vi "Edit Lock In (SubVI).vi"(8 "error in (no error)":errorcluster, 11 "Instrument parameters in":T1) -> (0 "error out":errorcluster, 3 "Instrument parameters out":T1)   [LabVIEW 2025, in "MyLockIn.lvlib"]
uses:
  MyLockIn.lvlib
panel:
  in  "Boolean":bool
  in  "Monitor sensitivity":bool
  in  "RESET?":bool
  in  "Auto Reserve":bool
  in  "Auto Phase":bool
  in  "Auto gain":bool
  out "Present value":string
  in  "Set new":bool
  in  "Read":bool
  in  "Select parameter":string(combo)="SENS"
  # "SETTINGS FOR LOCK-IN"
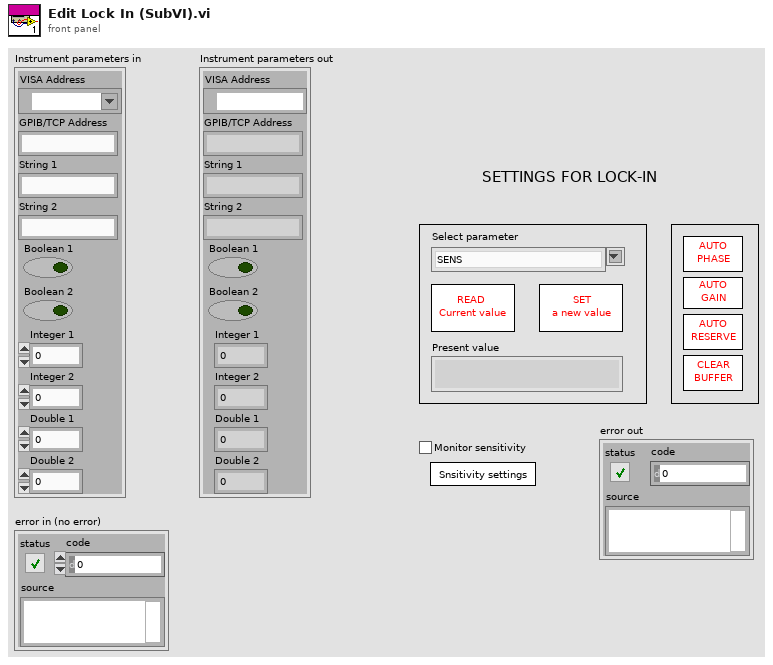
[diagram p1: front panel]
types:
  T1 = cluster{"VISA Address":refnum<visa-resource-name>, "GPIB/TCP Address":string, "String 1":string, "String 2":string, "Boolean 1":bool, "Boolean 2":bool, "Integer 1":i32, "Integer 2":i32, "Double 1":dbl, "Double 2":dbl}
  T2 = typedef "S2DS_Instrument parameters.ctl" = cluster{"VISA Address":refnum<visa-resource-name>, "GPIB/TCP Address":string, "String 1":string, "String 2":string, "Boolean 1":bool, "Boolean 2":bool, "Int 1":i32, "Int 2":i32, "Double 1":dbl, "Double 2":dbl}
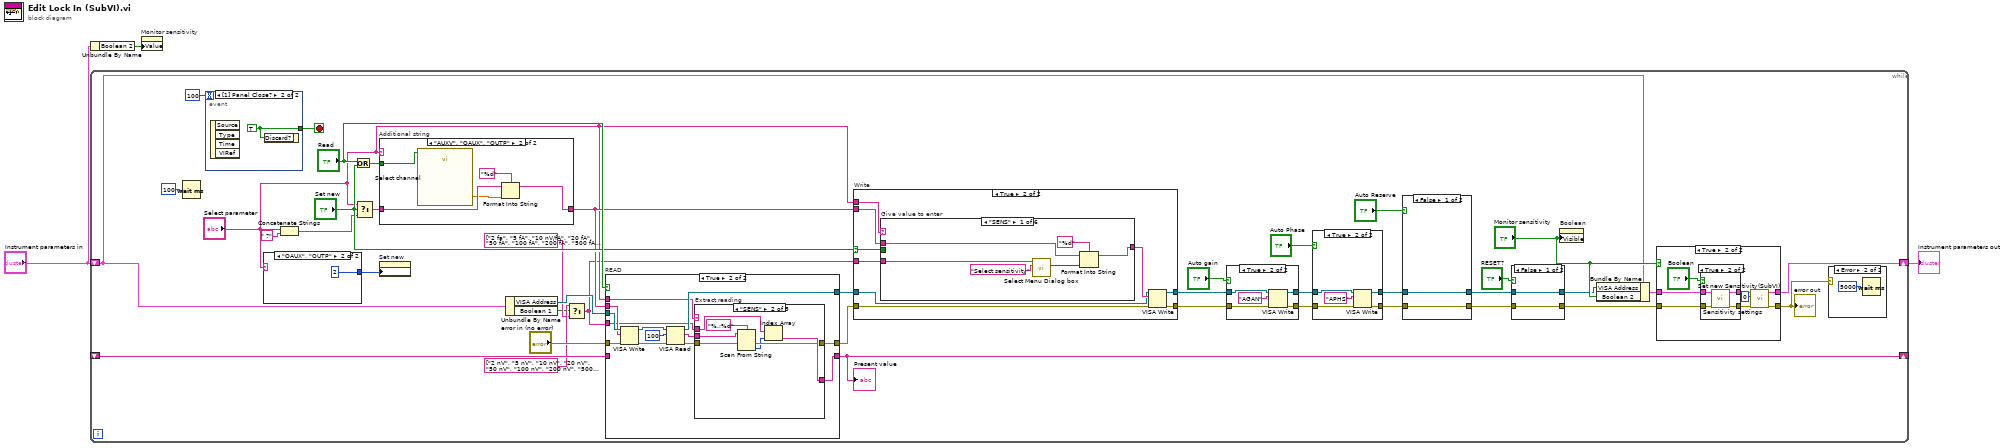
[diagram p0: block diagram]
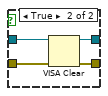
[diagram p4: hidden frame]
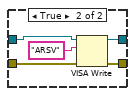
[diagram p5: hidden frame]
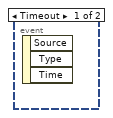
[diagram p9: hidden frame]
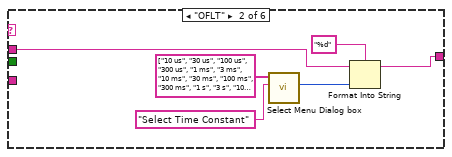
[diagram p11: hidden frame]
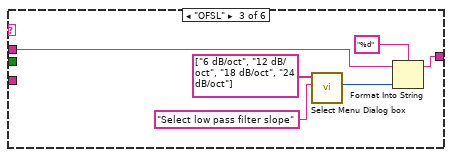
[diagram p12: hidden frame]
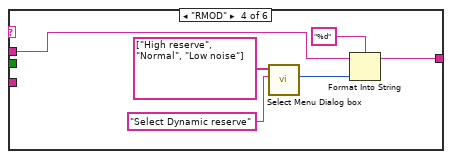
[diagram p13: hidden frame]
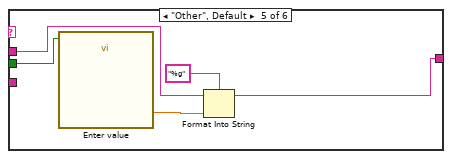
[diagram p14: hidden frame]
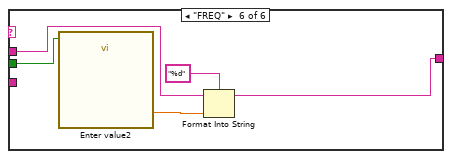
[diagram p15: hidden frame]
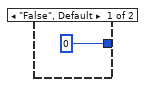
[diagram p16: hidden frame]
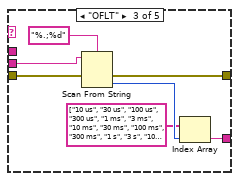
[diagram p19: hidden frame]
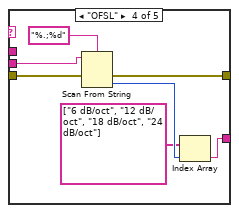
[diagram p20: hidden frame]
diagram:
  n1 = Unbundle By Name("Instrument parameters in") -> ("Boolean 2"=w1:bool)
  n2 = while {
    shift-right: [w37] -> _
    shift-left: _ -> [w36]
    shift-right: [w4] -> w3
    shift-left: "Instrument parameters in" -> [w6]
    stop <- w27 stop-if-true
    n3 = Wait (ms)(milliseconds to wait=u32 100) -> ()  [unwired: 1 out]
    n4 = event shown="[1] Panel Close?" {
      selector: _ -> [_ _]
      dyn-events: _ -> [_ _]
      timeout: 100 -> [_ _]
      tunnel: [_ w89] -> w27
      event Timeout {
        n5 = event-data() -> ()  [unwired: 1 in, 3 out]
      }
      event Panel Close? {
        w89 = TRUE ("Discard?")
        n6 = event-data() -> ()  [unwired: 1 in, 4 out]
        n7 = event-data("Discard?"=w89) -> ()  [unwired: 1 in, 1 out]
      }
    }
    n8 = case shown="\"OAUX\", \"OUTP\"" "Select parameter" {
      tunnel: [0 2] -> w38
      frame "False", Default {
      }
      frame "OAUX", "OUTP" {
      }
    }
    n9 = Concatenate Strings("Select parameter", " ?" ("string")) -> (w34:string)
    n10 = Or(x="Read", y="Set new") -> (x .or. y?=w40:bool)
    n11 = Select(t="Select parameter", s="Set new", f=w34) -> (s? t:f=w33:string)
    n12 = case "Additional string" shown="\"AUXV\", \"OAUX\", \"OUTP\"" "Select parameter" {
      tunnel: [w183 w184] -> w30
      tunnel: w33 -> [w183 w187]
      tunnel: w40 -> [_ w188]
      frame "False", Default {
      }
      frame "AUXV", "OAUX", "OUTP" {
        n13 = call "Select channel"("Enable"=w188) -> ("Select Channel"=w185:dbl)  [unwired: 16 in, 2 out]
        n14 = Format Into String(format string="%d", initial string=w187, w185) -> (resulting string=w184:string)  [unwired: 1 in, 1 out]
      }
    }
    n15 = property on="Set new" class="Bool"("DisabledEnum"=w38) -> ()  [unwired: 2 in, 2 out]
    n16 = Unbundle By Name(w6) -> ("VISA Address"=w44:refnum<visa-resource-name>, "Boolean 1"=w11:bool)
    n17 = Select(t=string[] ["2 nV", "5 nV", "10 nV", "20 nV", "50 nV", "100 nV", "200 nV", "500 nV", "1 uV", "2 uV", "5 uV", "10 uV", "20 uV", "50 uV", "100 uV", "200 uV", "500 uV", "1 mV", "2 mV", "5 mV", "10 mV", "20 mV", "50 mV", "100 mV", "200 mV", "500 mV", "1 V", "Error"], s=w11, f=string[] ["2 fa", "5 fA", "10 nV/fA", "20 fA", "50 fA", "100 fA", "200 fA", "500 fA", "1 pA", "2 pA", "5 pA", "10 pA", "20 pA", "50 pA", "100 pA", "200 pA", "500 pA", "1 nA", "2 nA", "5 nA", "10 nA", "20 nA", "50 nA", "100 nA", "200 nA", "500 nA", "1 uA", "Error"]) -> (s? t:f=w10:string[])
    n18 = case "READ" shown="True" "Read" {
      tunnel: w30 -> [_ w146]
      tunnel: w44 -> [w138 w149]
      tunnel: "error in (no error)" -> [w139 w148]
      tunnel: [w139 w142] -> w32
      tunnel: [w138 w147] -> w31
      tunnel: [w137 w145] -> w37
      tunnel: w36 -> [w137 _]
      tunnel: "Select parameter" -> [_ w144]
      tunnel: w10 -> [_ w140]
      frame False {
      }
      frame True {
        n19 = VISA Write(VISA resource name=w149, write buffer=w146, error in (no error)=w148) -> (VISA resource name out=w151:refnum<visa-resource-name>, error out=w150:errorcluster)  [unwired: 1 out]
        n20 = VISA Read(VISA resource name=w151, byte count=u32 100, error in (no error)=w150) -> (VISA resource name out=w147:refnum<visa-resource-name>, read buffer=w141:string, error out=w143:errorcluster)  [unwired: 1 out]
        n21 = case "Extract reading" shown="\"SENS\"" w144 {
          tunnel: [w154 w161 w168 w175 w182] -> w145
          tunnel: w143 -> [w153 w160 w167 w174 w181]
          tunnel: [w153 w159 w166 w173 w180] -> w142
          tunnel: w141 -> [w154 w157 w164 w171 w178]
          tunnel: w140 -> [_ w155 _ _ _]
          frame "False", Default {
          }
          frame "SENS" {
            n22 = Scan From String(format string="%.;%d", input string=w157, error in=w160) -> (error out=w159:errorcluster, output 1=w156:i32)  [unwired: 2 in, 2 out]
            n23 = Index Array(array=w155, index=w156) -> (element=w161:string)
          }
          frame "OFLT" {
            n24 = Scan From String(format string="%.;%d", input string=w164, error in=w167) -> (error out=w166:errorcluster, output 1=w163:i32)  [unwired: 2 in, 2 out]
            n25 = Index Array(array=string[] ["10 us", "30 us", "100 us", "300 us", "1 ms", "3 ms", "10 ms", "30 ms", "100 ms", "300 ms", "1 s", "3 s", "10 s", "30 s", "100 s", "300 s", "1 ks", "3 ks", "10 ks", "30 ks", "Error"], index=w163) -> (element=w168:string)
          }
          frame "OFSL" {
            n26 = Scan From String(format string="%.;%d", input string=w171, error in=w174) -> (error out=w173:errorcluster, output 1=w170:i32)  [unwired: 2 in, 2 out]
            n27 = Index Array(array=string[] ["6 dB/oct", "12 dB/oct", "18 dB/oct", "24 dB/oct"], index=w170) -> (element=w175:string)
          }
          frame "RMOD" {
            n28 = Scan From String(format string="%.;%d", input string=w178, error in=w181) -> (error out=w180:errorcluster, output 1=w177:i32)  [unwired: 2 in, 2 out]
            n29 = Index Array(array=string[] ["High reserve", "Normal", "Low noise"], index=w177) -> (element=w182:string)
          }
        }
      }
    }
    "Present value" <- w37
    n30 = case "Write" shown="True" "Set new" {
      selector: "Set new" -> [_ w93]
      tunnel: w32 -> [w91 w95]
      tunnel: [w91 w94] -> w25
      tunnel: w31 -> [w90 w97]
      tunnel: [w90 w96] -> w24
      tunnel: w30 -> [_ w99]
      tunnel: "Select parameter" -> [_ w100]
      tunnel: w10 -> [_ w92]
      frame False {
      }
      frame True {
        n31 = case "Give value to enter" shown="\"SENS\"" w100 {
          tunnel: w99 -> [w106 w112 w118 w124 w129 w134]
          tunnel: [w104 w110 w116 w122 w127 w132] -> w98
          tunnel: w93 -> [_ _ _ _ w126 w131]
          tunnel: w92 -> [w101 _ _ _ _ _]
          frame "SENS" {
            n32 = call "Select Menu Dialog box.vi"("Message in"="Select sensitivity", "Options in"=w101) -> ("Selected option number"=w103:i32)  [unwired: 9 in]
            n33 = Format Into String(format string="%d", initial string=w106, w103) -> (resulting string=w104:string)  [unwired: 1 in, 1 out]
          }
          frame "OFLT" {
            n34 = call "Select Menu Dialog box.vi"("Message in"="Select Time Constant", "Options in"=string[] ["10 us", "30 us", "100 us", "300 us", "1 ms", "3 ms", "10 ms", "30 ms", "100 ms", "300 ms", "1 s", "3 s", "10 s", "30 s", "100 s", "300 s", "1 ks", "3 ks", "10 ks", "30 ks", "Error"] ("array")) -> ("Selected option number"=w109:i32)  [unwired: 9 in]
            n35 = Format Into String(format string="%d", initial string=w112, w109) -> (resulting string=w110:string)  [unwired: 1 in, 1 out]
          }
          frame "OFSL" {
            n36 = call "Select Menu Dialog box.vi"("Message in"="Select low pass filter slope", "Options in"=string[] ["6 dB/oct", "12 dB/oct", "18 dB/oct", "24 dB/oct"] ("array")) -> ("Selected option number"=w115:i32)  [unwired: 9 in]
            n37 = Format Into String(format string="%d", initial string=w118, w115) -> (resulting string=w116:string)  [unwired: 1 in, 1 out]
          }
          frame "RMOD" {
            n38 = call "Select Menu Dialog box.vi"("Message in"="Select Dynamic reserve", "Options in"=string[] ["High reserve", "Normal", "Low noise"] ("array")) -> ("Selected option number"=w121:i32)  [unwired: 9 in]
            n39 = Format Into String(format string="%d", initial string=w124, w121) -> (resulting string=w122:string)  [unwired: 1 in, 1 out]
          }
          frame "Other", Default {
            n40 = call "Enter value"("Enable"=w126) -> ("Value"=w125:dbl)  [unwired: 16 in, 2 out]
            n41 = Format Into String(format string="%g", initial string=w129, w125) -> (resulting string=w127:string)  [unwired: 1 in, 1 out]
          }
          frame "FREQ" {
            n42 = call "Enter value2"("Enable"=w131) -> ("Frequency"=w130:dbl)  [unwired: 16 in, 2 out]
            n43 = Format Into String(format string="%d", initial string=w134, w130) -> (resulting string=w132:string)  [unwired: 1 in, 1 out]
          }
        }
        n44 = VISA Write(VISA resource name=w97, write buffer=w98, error in (no error)=w95) -> (VISA resource name out=w96:refnum<visa-resource-name>, error out=w94:errorcluster)  [unwired: 1 out]
      }
    }
    n45 = case shown="True" "Auto gain" {
      tunnel: [w82 w85] -> w22
      tunnel: w25 -> [w82 w86]
      tunnel: w24 -> [w81 w87]
      tunnel: [w81 w83] -> w21
      frame False {
      }
      frame True {
        n46 = VISA Write(VISA resource name=w87, write buffer="AGAN", error in (no error)=w86) -> (VISA resource name out=w83:refnum<visa-resource-name>, error out=w85:errorcluster)  [unwired: 1 out]
      }
    }
    n47 = case shown="True" "Auto Phase" {
      tunnel: [w75 w78] -> w19
      tunnel: w22 -> [w75 w79]
      tunnel: w21 -> [w74 w80]
      tunnel: [w74 w76] -> w18
      frame False {
      }
      frame True {
        n48 = VISA Write(VISA resource name=w80, write buffer="APHS", error in (no error)=w79) -> (VISA resource name out=w76:refnum<visa-resource-name>, error out=w78:errorcluster)  [unwired: 1 out]
      }
    }
    n49 = case shown="False" "Auto Reserve" {
      tunnel: [w68 w71] -> w15
      tunnel: w19 -> [w68 w72]
      tunnel: w18 -> [w67 w73]
      tunnel: [w67 w69] -> w16
      frame False {
      }
      frame True {
        n50 = VISA Write(VISA resource name=w73, write buffer="ARSV", error in (no error)=w72) -> (VISA resource name out=w69:refnum<visa-resource-name>, error out=w71:errorcluster)  [unwired: 1 out]
      }
    }
    n51 = case shown="False" "RESET?" {
      tunnel: [w62 w65] -> w14
      tunnel: w15 -> [w62 w66]
      tunnel: w16 -> [w61 w64]
      tunnel: [w61 w63] -> w7
      frame False {
      }
      frame True {
        n52 = VISA Clear(VISA resource name=w64, error in (no error)=w66) -> (VISA resource name out=w63:refnum<visa-resource-name>, error out=w65:errorcluster)
      }
    }
    n53 = property on="Boolean" class="Bool"("Visible"="Monitor sensitivity") -> ()  [unwired: 2 in, 2 out]
    n54 = Bundle By Name(cluster=w6, "VISA Address"=w7, "Boolean 2"="Monitor sensitivity") -> (w5:T2)
    n55 = case shown="True" "Monitor sensitivity" {
      tunnel: w14 -> [w46 w49]
      tunnel: [w46 w51] -> w8
      tunnel: w5 -> [w45 w53]
      tunnel: [w45 w50] -> w4
      frame False {
      }
      frame True {
        n56 = case shown="True" "Boolean" {
          tunnel: [w56 w60] -> w52
          tunnel: w53 -> [w56 w59]
          tunnel: w49 -> [w55 w58]
          tunnel: [w55 w57] -> w48
          frame False {
          }
          frame True {
            n57 = call "Sensitivity settings.vi"("error in"=w58, "Instrument parameters in"=w59) -> ("error IO"=w57:errorcluster, "Instrument parameters out"=w60:T1)  [unwired: 8 in]
          }
        }
        n58 = call "Set new Sensitivity(SubVI).vi"("error in (no error)"=w48, "Numeric"=0, "Instrument parameters in"=w52) -> ("error out"=w51:errorcluster, "Instrument parameters out"=w50:T2)  [unwired: 6 in, 1 out]
      }
    }
    "error out" <- w8
    n59 = case shown="Error" w8 {
      frame No Error {
      }
      frame Error {
        n60 = Wait (ms)(milliseconds to wait=u32 5000) -> ()  [unwired: 1 out]
      }
    }
  }
  "Instrument parameters out" <- w3
  n61 = property on="Monitor sensitivity" class="Bool (strict)"("Value"=w1) -> ()  [unwired: 2 in, 2 out]
